vi "MD5Checksum File.vi"(8 "error in (no error)":errorcluster, 11 "Path":path) -> (0 "error out":errorcluster, 3 "MD5 message-digest":string)   [LabVIEW 2010]
doc: "Computes the MD5 message-digest of a file. The MD5 message-digest is a 128-bit number displayed in lowercase hexadecimal format."
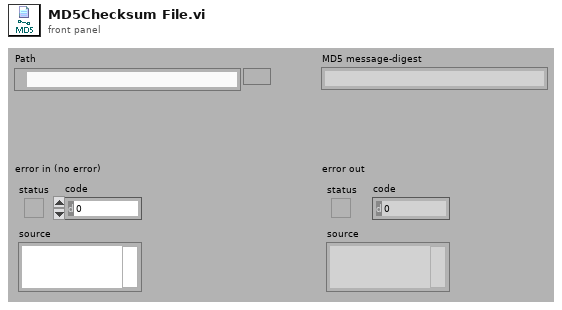
[diagram p1: front panel]
types:
  T1 = enum16{"open", "replace", "create", "open or create", "replace or create", "replace or create with confirmation"}
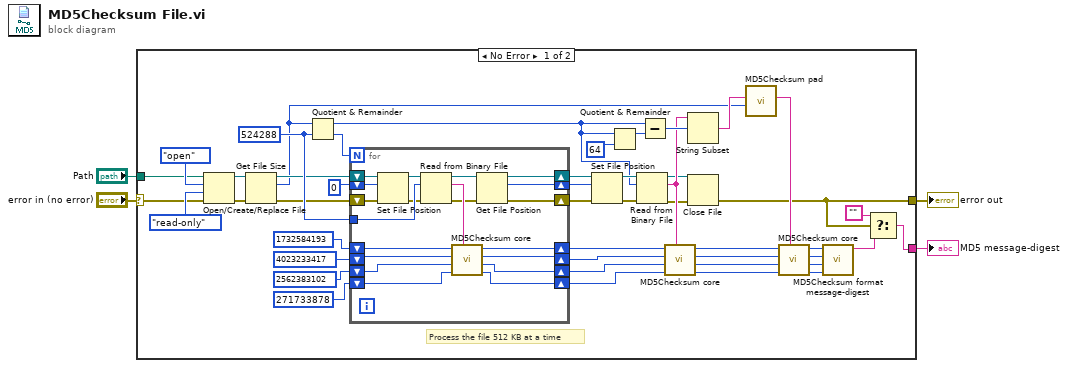
[diagram p0: block diagram]
diagram:
  n1 = case shown="No Error" "error in (no error)" {
    selector: "error in (no error)" -> [w15 w71]
    tunnel: "Path" -> [w14 _]
    tunnel: [w6 _] -> w3
    tunnel: [w7 w71] -> w2
    frame No Error {
      w24 = 524288 ("y")
      # "Process the file 512 KB at a time"
      n2 = Open/Create/Replace File(file path (use dialog)=w14, error in=w15, operation (0:open)=T1."open", access (0:read/write)=enum16{"read/write", "read-only", "write-only"}."read-only") -> (refnum out=w12:refnum<file>, error out=w13:errorcluster)  [unwired: 2 in, 1 out]
      n3 = Get File Size(file=w12, error in=w13) -> (refnum out=w10:refnum<file>, size (in bytes)=w9:i64, 0:w11:errorcluster)
      n4 = Quotient & Remainder(x=w9, y=w24) -> (x-y*floor(x/y)=w18:i64, floor(x/y)=w50:i64)
      n5 = for {
        N: w50 -> [_]
        shift-right: [w64] -> w45
        shift-left: u32 1732584193 ("s1") -> [w69]
        shift-right: [w63] -> w44
        shift-left: u32 4023233417 ("s2") -> [w68]
        shift-right: [w62] -> w43
        shift-left: u32 2562383102 ("s3") -> [w67]
        shift-right: [w61] -> w42
        shift-left: u32 271733878 ("s4") -> [w66]
        shift-right: [w51] -> w39
        shift-left: i64 0 ("offset") -> [w59]
        tunnel: w24 -> [w58]
        shift-right: [w60] -> w40
        shift-left: w10 -> [w70]
        shift-right: [w56] -> w21
        shift-left: w11 -> [w57]
        n6 = Set File Position(offset (in bytes) (0)=w59, refnum=w70, error in=w57) -> (refnum out=w55:refnum<file>, error out=w54:errorcluster)  [unwired: 1 in]
        n7 = Read from Binary File(8:w54, 10:w58, 11:w55) -> (0:w52:errorcluster, 2:w65:string, 3:w53:refnum<file>)  [unwired: 3 in, 1 out]
        n8 = call <vilib>:"MD5Checksum core.vi"("Input String"=w65, "s4 in"=w66, "s3 in"=w67, "s2 in"=w68, "s1 in"=w69) -> ("s4 out"=w61:u32, "s3 out"=w62:u32, "s2 out"=w63:u32, "s1 out"=w64:u32)  [unwired: 3 in]
        n9 = Get File Position(4:w52, 7:w53) -> (0:w56:errorcluster, 2:w51:i64, 3:w60:refnum<file>)
      }
      n10 = Set File Position(offset (in bytes) (0)=w39, refnum=w40, error in=w21) -> (refnum out=w20:refnum<file>, error out=w19:errorcluster)  [unwired: 1 in]
      n11 = Quotient & Remainder(x=w18, y=64) -> (x-y*floor(x/y)=w37:i64)  [unwired: 1 out]
      n12 = Read from Binary File(8:w19, 10:w18, 11:w20) -> (0:w22:errorcluster, 2:w25:string, 3:w23:refnum<file>)  [unwired: 3 in, 1 out]
      n13 = Subtract(x=w18, y=w37) -> (x-y=w36:i64)
      n14 = call <vilib>:"MD5Checksum core.vi"("Input String"=w25, "s4 in"=w42, "s3 in"=w43, "s2 in"=w44, "s1 in"=w45) -> ("s4 out"=w31:u32, "s3 out"=w32:u32, "s2 out"=w33:u32, "s1 out"=w34:u32)  [unwired: 3 in]
      n15 = String Subset(string=w25, offset (0)=w36) -> (substring=w35:string)  [unwired: 1 in]
      n16 = Close File(refnum=w23, error in=w22) -> (error out=w7:errorcluster)  [unwired: 1 out]
      n17 = call <vilib>:"MD5Checksum pad.vi"("Message String Length (bytes)"=w9, "Last Part of Message String"=w35) -> ("Padding"=w30:string)  [unwired: 9 in]
      n18 = call <vilib>:"MD5Checksum core.vi"("Input String"=w30, "s4 in"=w31, "s3 in"=w32, "s2 in"=w33, "s1 in"=w34) -> ("s4 out"=w26:u32, "s3 out"=w27:u32, "s2 out"=w28:u32, "s1 out"=w29:u32)  [unwired: 3 in]
      n19 = call <vilib>:"MD5Checksum format message-digest.vi"("s4"=w26, "s3"=w27, "s2"=w28, "s1"=w29) -> ("MD5 message-digest"=w8:string)  [unwired: 7 in]
      n20 = Select(t="", s=w7, f=w8) -> (s? t:f=w6:string)
    }
    frame Error {
    }
  }
  "MD5 message-digest" <- w3
  "error out" <- w2
